vi "FlatToRichGreeter_req.vi"(5 "OutputClusterType":T1, 11 "InputCluster":T2) -> (3 "OutputCluster":T1)   [LabVIEW 2019, in "Generated_server.lvlib"]
uses:
  Generated_server.lvlib
  Greeter_req_Flat.ctl
  Greeter_MessageA_Flat.ctl
  Greeter_req.ctl
  Greeter_req_req_oneof/Greeter_req_req_oneof.lvclass
  Greeter_MessageA_oneof_a/Greeter_MessageA_oneof_a.lvclass/Greeter_MessageA_oneof_a.ctl
  Greeter_req_req_oneof/Greeter_req_req_oneof.lvclass/Greeter_req_req_oneof.ctl
  Greeter_MessageA_oneof_a/Setdata_a1.vi
  Greeter_MessageA_oneof_a/Setdata_a2.vi
  Greeter_MessageA_oneof_a/GetFieldFromProtobufIndexGreeter_MessageA_oneof_a.vi
  Greeter_MessageA_oneof_a/Greeter_MessageA_oneof_a.lvclass
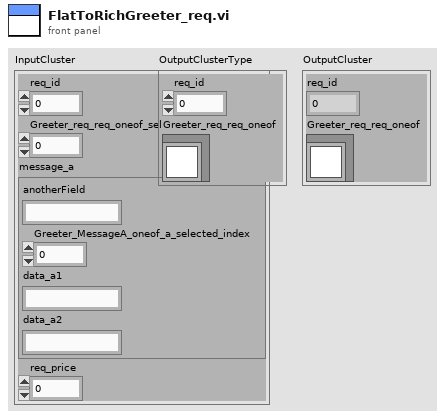
[diagram p1: front panel]
types:
  T1 = typedef "Generated_server.lvlib/Greeter_req.ctl" = cluster{"req_id":i32, "Greeter_req_req_oneof":refnum<class "Greeter_req_req_oneof.lvclass">}
  T2 = typedef "Generated_server.lvlib/Greeter_req_Flat.ctl" = cluster{"req_id":i32, "Greeter_req_req_oneof_selected_index":i32, "message_a":T3, "req_price":dbl}
  T3 = typedef "Generated_server.lvlib/Greeter_MessageA_Flat.ctl" = cluster{"anotherField":string, "Greeter_MessageA_oneof_a_selected_index":i32, "data_a1":string, "data_a2":string}
  T4 = typedef "Generated_server.lvlib/Greeter_MessageA.ctl" = cluster{"anotherField":string, "Greeter_MessageA_oneof_a":refnum<class "Greeter_MessageA_oneof_a.lvclass">}
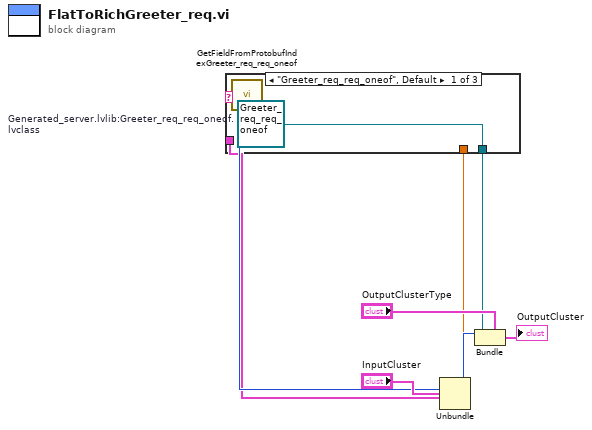
[diagram p0: block diagram]
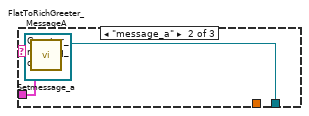
[diagram p2: hidden frame]
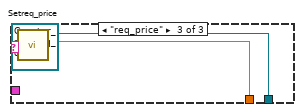
[diagram p3: hidden frame]
diagram:
  n1 = Unbundle "Unbundle"("InputCluster") -> ("req_id"=w6:i32, "Greeter_req_req_oneof_selected_index"=w5:i32, "message_a"=w2:T3, "req_price"=w1:dbl)
  n2 = call "GetFieldFromProtobufIndexGreeter_req_req_oneof.vi"("protobuf index"=w5) -> ("oneof field name"=w4:string)
  n3 = case "Greeter_req_req_oneof" shown="\"Greeter_req_req_oneof\", Default" w4 {
    tunnel: [w10 w12 w16] -> w3
    tunnel: w2 -> [_ w14 _]
    tunnel: w1 -> [_ _ w17]
    frame "Greeter_req_req_oneof", Default {
      w10 = refnum<class "Greeter_req_req_oneof.lvclass"> refnum  # Generated_server.lvlib:Greeter_req_req_oneof.lvclass
    }
    frame "message_a" {
      n4 = call "FlatToRichGreeter_MessageA.vi"("InputCluster"=w14) -> ("OutputCluster"=w13:T4)  [unwired: 10 in]
      n5 = call "Setmessage_a.vi"("Set_Val"=w13, "OneOfTemplate in"=refnum<class "Greeter_req_req_oneof.lvclass"> refnum) -> ("OneOfTemplate out"=w12:refnum<class "Greeter_req_req_oneof.lvclass">)  [unwired: 8 in, 1 out]
    }
    frame "req_price" {
      n6 = call "Setreq_price.vi"("Set_Val"=w17, "OneOfTemplate in"=refnum<class "Greeter_req_req_oneof.lvclass"> refnum) -> ("OneOfTemplate out"=w16:refnum<class "Greeter_req_req_oneof.lvclass">)  [unwired: 8 in, 1 out]
    }
  }
  n7 = Bundle "Bundle"(cluster="OutputClusterType", "req_id"=w6, "Greeter_req_req_oneof"=w3) -> (→"OutputCluster":T1)
